vi "Graph Prep.vi"(0 "V_PIdata":dbl[](array[numeric]), 1 "InstDataCluster":T2, 2 "AveDataCluster":T2, 3 "Enable Graphs":bool, 4 "GraphTab":enum32{"Page 1", "Page 2"}(ring), 5 "Pres_PIdata":dbl[](array[numeric]), 7 "CMD_PIdata":dbl[](array[numeric]), 9 "VSig":dbl format="%#_13g", 11 "PresSig":dbl format="%#_13g", 12 "CMDSig":dbl format="%#_13g", 13 "Controller?":bool, 14 "TolBounds":dbl[][](array[numeric]), 15 "CommandCluster":T1) -> ()   [LabVIEW 2013]
uses:
  TypeDef/DataCluster.ctl
  TypeDef/Command Cluster.ctl
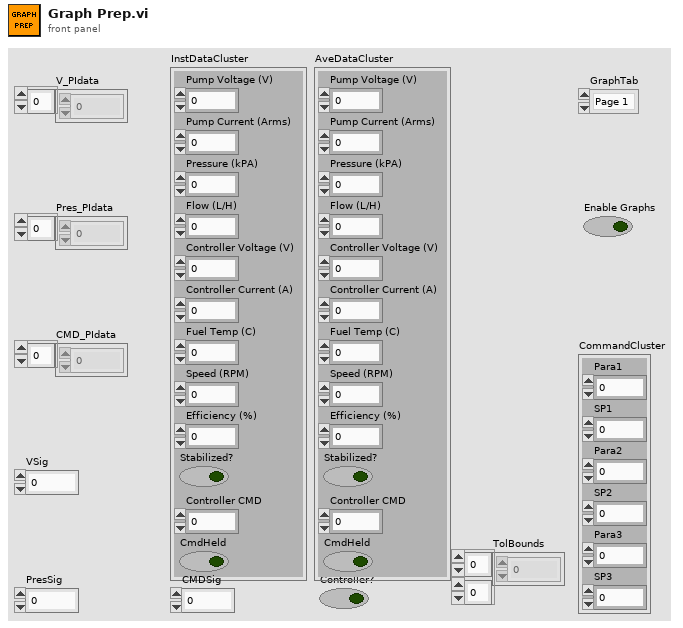
[diagram p1: front panel]
types:
  T1 = typedef "Command Cluster.ctl" = cluster{"Para1":i32, "SP1":dbl, "Para2":i32, "SP2":dbl, "Para3":i32, "SP3":dbl}
  T2 = typedef "DataCluster.ctl" = cluster{"Pump Voltage (V)":dbl, "Pump Current (Arms)":dbl, "Pressure (kPA)":dbl, "Flow (L/H)":dbl, "Controller Voltage (V)":dbl, "Controller Current (A)":dbl, "Fuel Temp (C)":dbl, "Speed (RPM)":dbl, "Efficiency (%)":dbl, "Stabilized?":bool, "Controller CMD":dbl, "CmdHeld":bool}
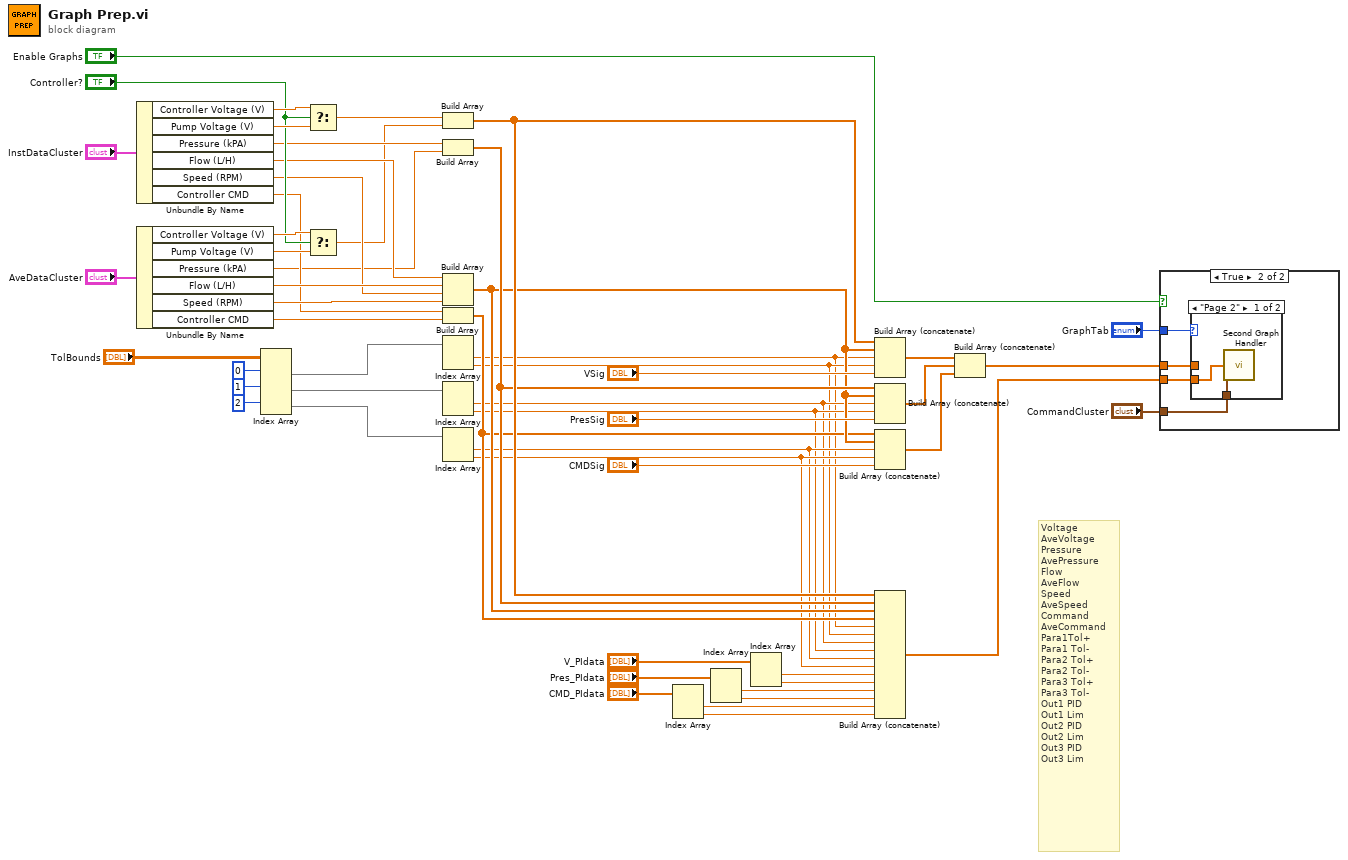
[diagram p0: block diagram]
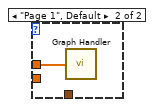
[diagram p3: hidden frame]
diagram:
  # "Voltage\nAveVoltage\nPressure\nAvePressure\nFlow\nAveFlow\nSpeed\nAveSpeed\nCommand\nAveCommand\nPara1Tol+\nPara1 Tol-\nPara2 Tol+\nPara2 Tol-\nPara3 Tol+\nPara3 Tol-\nOut1 PID\nOut1 Lim\nOut2 PID\nOut2 Lim\nOut3 PID\nOut3 Lim"
  n1 = Unbundle By Name("InstDataCluster") -> ("Controller Voltage (V)"=w49:dbl, "Pump Voltage (V)"=w50:dbl, "Pressure (kPA)"=w31:dbl, "Flow (L/H)"=w41:dbl, "Speed (RPM)"=w38:dbl, "Controller CMD"=w33:dbl)
  n2 = Unbundle By Name("AveDataCluster") -> ("Controller Voltage (V)"=w52:dbl, "Pump Voltage (V)"=w51:dbl, "Pressure (kPA)"=w32:dbl, "Flow (L/H)"=w40:dbl, "Speed (RPM)"=w39:dbl, "Controller CMD"=w34:dbl)
  n3 = Index Array(array="TolBounds", index (row) #1=0 ("index (row)"), index (row) #2=1 ("index (row)"), index (row) #3=2 ("index (row)")) -> (element #1=w5:dbl[], element #2=w6:dbl[], element #3=w9:dbl[])  [unwired: 3 in]
  n4 = Select(t=w49, s="Controller?", f=w50) -> (s? t:f=w30:dbl)
  n5 = Select(t=w52, s="Controller?", f=w51) -> (s? t:f=w29:dbl)
  n6 = Build Array(w30, w29) -> (w28:dbl[])
  n7 = Build Array(w31, w32) -> (w27:dbl[])
  n8 = Build Array(w41, w40, w38, w39) -> (w26:dbl[])
  n9 = Build Array(w33, w34) -> (w25:dbl[])
  n10 = Index Array(array=w5) -> (element #1=w1:dbl, element #2=w2:dbl)  [unwired: 2 in]
  n11 = Index Array(array=w6) -> (element #1=w3:dbl, element #2=w4:dbl)  [unwired: 2 in]
  n12 = Index Array(array=w9) -> (element #1=w7:dbl, element #2=w8:dbl)  [unwired: 2 in]
  n13 = Index Array(array="CMD_PIdata") -> (element #1=w20:dbl, element #2=w19:dbl)  [unwired: 2 in]
  n14 = Index Array(array="Pres_PIdata") -> (element #1=w22:dbl, element #2=w21:dbl)  [unwired: 2 in]
  n15 = Index Array(array="V_PIdata") -> (element #1=w24:dbl, element #2=w23:dbl)  [unwired: 2 in]
  n16 = Build Array (concatenate)(w28, w26, w1, w2, "VSig") -> (w47:dbl[])
  n17 = Build Array (concatenate)(w27, w26, w3, w4, "PresSig") -> (w46:dbl[])
  n18 = Build Array (concatenate)(w25, w26, w7, w8, "CMDSig") -> (w45:dbl[])
  n19 = Build Array (concatenate)(w28, w27, w26, w25, w1, w2, w3, w4, w7, w8, w24, w23, w22, w21, w20, w19) -> (w17:dbl[])
  n20 = Build Array (concatenate)(w47, w46, w45) -> (w18:dbl[])
  n21 = case shown="True" "Enable Graphs" {
    tunnel: w18 -> [_ w58]
    tunnel: w17 -> [_ w57]
    tunnel: "GraphTab" -> [_ w56]
    tunnel: "CommandCluster" -> [_ w55]
    frame False {
    }
    frame True {
      n22 = case shown="\"Page 2\"" w56 {
        tunnel: w58 -> [_ w61]
        tunnel: w57 -> [w60 _]
        tunnel: w55 -> [w59 _]
        frame "Page 2" {
          n23 = call "Second Graph Handler.vi"("Data"=w60, "CommandCluster"=w59) -> ()  [unwired: 14 in]
        }
        frame "Page 1", Default {
          n24 = call "Graph Handler.vi"("Data"=w61) -> ()  [unwired: 15 in]
        }
      }
    }
  }
